vi "MM Sample Test.vi"(8 "error in":errorcluster, 11 "objects IN":T2) -> (0 "error out":errorcluster, 3 "objects OUT":T2)   [LabVIEW 2011]
uses:
  Controls/Class Objects.ctl
  Modules/File/Configuration/Configuration.lvclass
  Modules/Hardware/PID/PID.lvclass
  Modules/Hardware/Power Supply/Power Supply.lvclass
  Modules/Hardware/Mass Flow Controller/Mass Flow Controller.lvclass
  Modules/Hardware/Valve Controller/Valve Controller.lvclass
  Modules/Hardware/Multimeter/Multimeter.lvclass
  Modules/Hardware/Vapour Generator/Vapour Generator.lvclass
  Modules/File/TDMS/TDMS.lvclass
  Modules/Hardware/Aalborg GFC17/Flow Rate.ctl
  Controls/User Interface Action.ctl
  Functional Global Data/Device Params Global.ctl
  Modules/File/TDMS/Data Type.ctl
  Controls/TDMS File Handling.ctl
  Modules/Hardware/Aalborg GFC17/Aalborg GFC17.lvclass
panel:
  in  "MFC Flow Rate":T1 caption="Flow Rate" min=0.0 max=200.0 scale=0.0..200.0
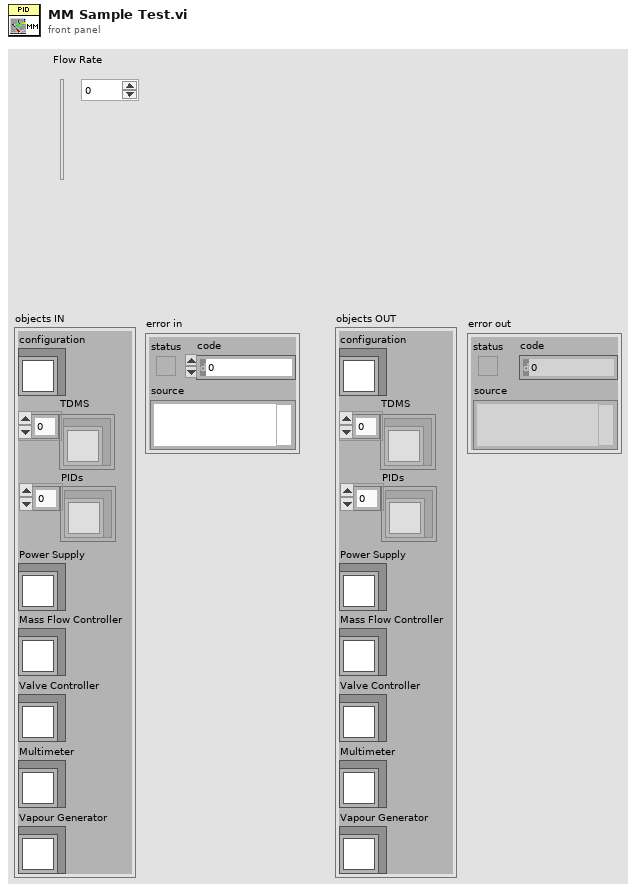
[diagram p1: front panel]
types:
  T1 = typedef "Aalborg GFC17.lvclass/Flow Rate.ctl" = dbl
  T2 = typedef "Class Objects.ctl" = cluster{"configuration":refnum<class "Configuration.lvclass">, "TDMS":refnum<class "TDMS.lvclass">[], "Power Supply":refnum<class "Power Supply.lvclass">, "Mass Flow Controller":refnum<class "Mass Flow Controller.lvclass">, "Valve Controller":refnum<class "Valve Controller.lvclass">, "Multimeter":refnum<class "Multimeter.lvclass">, "Vapour Generator":refnum<class "Vapour Generator.lvclass">, "PIDs":refnum<class "PID.lvclass">[]}
  T3 = typedef "User Interface Action.ctl" = enum16{"Initialize", "Data Acquisition Disable", "Data View Disable", "Sample Set", "Sample Set 2D Data", "Sample Set x0 & dx", "Sample Add", "Sample Set Cursor", "Sample Set Offset & Multiplier", "Sample Set Axis Labels", "Sample Parameters Disabled", "Sample Parameters Update", "Run Update", "Run Set Offset & Multiplier", "Run Set Axis Labels", "Run Set Cursor", "Run Set Disabled", "Run Parameters Update", "Run Parameters Disabled", "Run Number Set", "Run Number Set Range", "Run Number Set Disabled", "Sample Number Set", "Sample Number Set Range", "Notes Set Value", "Update Plot", "Set Plot Parameters", "Update Concentration Plot", "Time Set", "Clear DAQ Display", "Clear Analysis Display", "Status Bar Set", "Progress Bar Set", "Display Mode Set", "Experiment Type Set", "Analysis Plot Average Set", "Stop"}
  T4 = typedef "Device Params Global.ctl" = enum16{"Initialize", "Get Device Settings", "Get Device Connections", "Set Device Settings", "Set Device Connections", "Get All Device Properties"}
  T5 = typedef "TDMS.lvclass/Data Type.ctl" = enum16{"I16", "Double", "Waveform"}
  T6 = typedef "TDMS File Handling.ctl" = enum16{"Add TDMS File", "Get Active TDMS File", "Set Active TDMS File", "Set Active TDMS File Index"}
  T7 = typedef "Device Settings.ctl" = cluster{"PID":cluster{"B-M PID":T8, "INL PID":T9}, "Power Supply":cluster{"Source Value":dbl, "Source Value Units":T10, "Source Mode":T11, "Limits":T12, "Output":bool}, "Mass Flow Controller":cluster{"MFC Flow Rate":dbl, "MFC Valve Status":T15}, "Valve Controller":cluster{"Valve Assembly":T16}, "Multimeter":cluster{"Agilent 3458A":cluster{"Measurement Configuration":T18, "Measurement Integration":T19}}, "Vapour Generator":cluster{"Owlstone Permeation Tube":T20, "Owlstone GEN-SYS Setpoints":T22}}
  T8 = typedef "Baseline Mocon piD-Tech plus.lvclass/Settings.ctl" = cluster{"Detector Sampling Frequency":dbl}
  T9 = typedef "INL PID.lvclass/Settings.ctl" = cluster{"Sampling Frequency":dbl, "Integration Time":dbl, "Integration Periods":u8, "Grid Voltage":dbl}
  T10 = typedef "Power Supply.lvclass/Source Units.ctl" = enum16{"volts", "millivolts", "microvolts", "amps", "milliamps", "microamps", "nanoamps"}
  T11 = typedef "Power Supply.lvclass/Source Mode.ctl" = enum16{"Volts", "Current"}
  T12 = typedef "Power Supply.lvclass/Protection Limits.ctl" = cluster{"Voltage Limit":dbl, "Voltage Limit Units":T13, "Current Limit":dbl, "Current Limit Units":T14, "Voltage Trip/Cmpl":dbl, "Voltage Trip/Cmpl Units":T13, "Current Trip/Cmpl":dbl, "Current Trip/Cmpl Units":T14}
  T13 = typedef "Power Supply.lvclass/Voltage Units.ctl" = enum16{"volts", "millivolts", "microvolts"}
  T14 = typedef "Power Supply.lvclass/Current Units.ctl" = enum16{"amps", "milliamps", "microamps", "nanoamps"}
  T15 = typedef "Mass Flow Controller.lvclass/Valve Status.ctl" = enum16{"Open", "Closed"}
  T16 = typedef "Valve Controller.lvclass/Valve Assembly.ctl" = cluster{"Valve 1":T17, "Valve 2":T17, "Valve 3":T17, "Valve 4":T17, "Valve 5":T17}
  T17 = typedef "Valve Controller.lvclass/Status.ctl" = u16
  T18 = typedef "Agilent 3458A.lvclass/Measurement Configuration.ctl" = cluster{"Function":enum16{"DC Voltage", "AC Voltage", "AC + DC Voltage", "DC Current", "AC Current", "AC + DC Current", "2-Wire Resistance", "4-Wire Resistance", "Frequency", "Period", "Direct Sampling DC", "Direct Sampling AC", "Sub-Sampling DC", "Sub-Sampling AC"}, " Manual Resolution":enum16{"4.5", "5.5", "6.5", "7.5", "8.5"}, "Frequency Source":enum16{"AC + DC Current", "AC + DC Voltage", "AC Current", "AC Voltage"}, "Auto Range":enum16{"OFF", "ON", "ONCE"}}
  T19 = typedef "Agilent 3458A.lvclass/Measurement Integration.ctl" = cluster{"Power Line Cycles":dbl}
  T20 = typedef "Owlstone GEN-SYS.lvclass/Permeation Tube.ctl" = cluster{"Tube":T21, "Molecular Weight":dbl, "Calibration Temperature\n(Celcius)":i32, "Permeation Rate \n(ng/min)":i32}
  T21 = typedef "Owlstone GEN-SYS.lvclass/Permeation Tube Gas.ctl" = enum16{"Isobutylene 27 Nov 2012", "Ammonia 29 Sep 2012", "DMMP Tube A 3 July 2014", "DMMP Tube B 3 July 2014"}
  T22 = typedef "Owlstone GEN-SYS.lvclass/Gen-Sys Setpoints.ctl" = cluster{"OVG-4":cluster{"Oven Temperature":i32, "Sample Flow Rate":i32, "Split Flow Status":u16, "Split Flow Rate":i32}, "OHG-4":cluster{"Wet Air Flow":i32}}
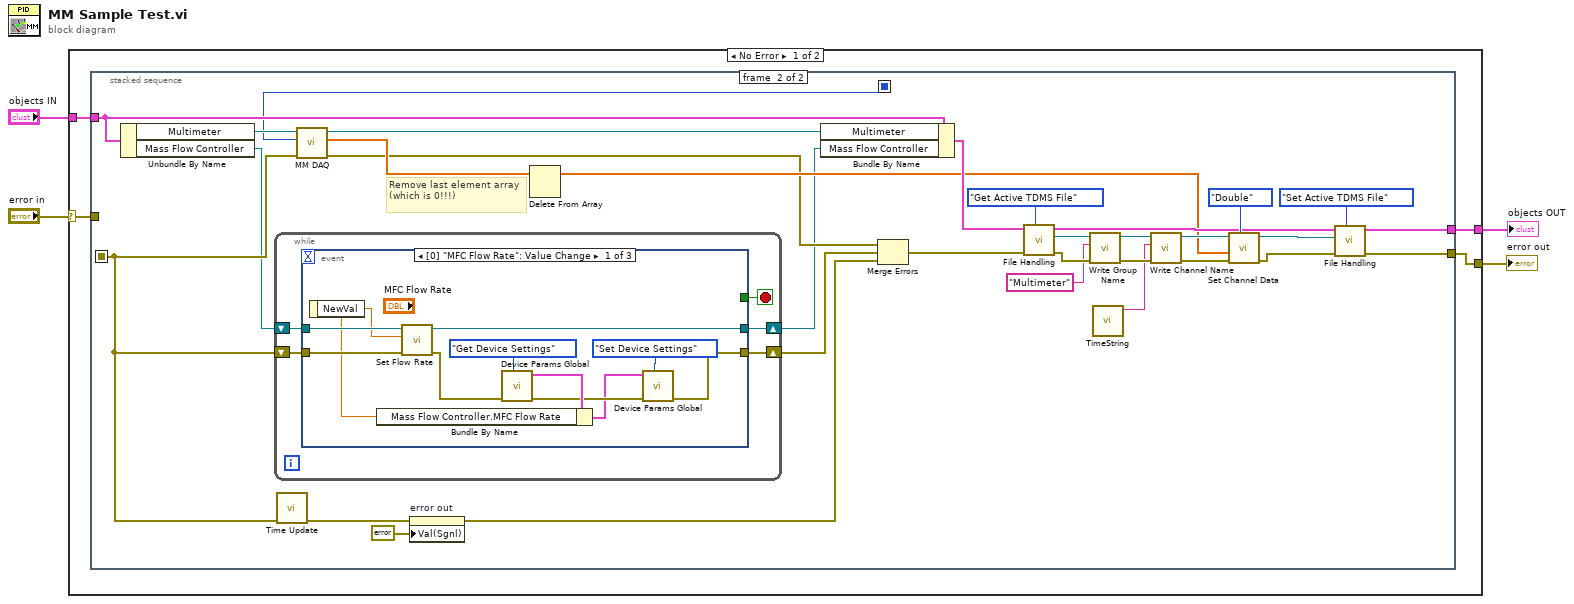
[diagram p0: block diagram]
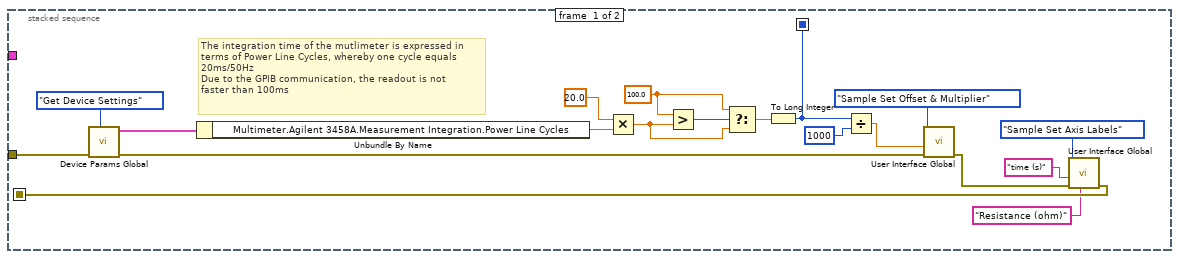
[diagram p2: hidden frame]
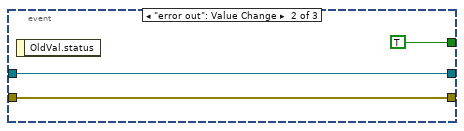
[diagram p3: hidden frame]
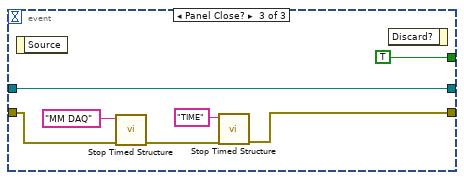
[diagram p4: hidden frame]
diagram:
  n1 = case shown="No Error" "error in" {
    selector: "error in" -> [w5 w86]
    tunnel: "objects IN" -> [w8 w87]
    tunnel: [w6 w87] -> w3
    tunnel: [w7 w86] -> w1
    frame No Error {
      n2 = stacked-sequence {
        seq-local: [w16 _] -> [_ w39]
        seq-local: [w10 _] -> [_ w36]
        tunnel: w8 -> [_ w59]
        tunnel: [_ w52] -> w7
        tunnel: [_ w50] -> w6
        tunnel: w5 -> [w25 _]
        frame #0 {
          w21 = 100.0 ("x")
          # "The integration time of the mutlimeter is expressed in\nterms of Power Line Cycles, whereby one cycle equals\n20ms/50Hz\nDue to the GPIB communication, the readout is not\nfaster than 100ms"
          n3 = call "Device Params Global.vi"("action"=Device_Params_Global."Get Device Settings", "error in"=w25) -> ("error out"=w17:errorcluster, "Device Settings OUT"=w26:T7)  [unwired: 7 in, 1 out]
          n4 = Unbundle By Name(w26) -> ("Multimeter.Agilent 3458A.Measurement Integration.Power Line Cycles"=w24:dbl)
          n5 = Multiply(x=20.0, y=w24) -> (x*y=w20:dbl)
          n6 = Greater?(x=w21, y=w20) -> (0:w22:bool)
          n7 = Select(t=w21, s=w22, f=w20) -> (s? t:f=w19:dbl)
          n8 = To Long Integer(number=w19) -> (32bit integer=w16:i32)
          n9 = Divide(x=w16, y=1000) -> (x/y=w14:dbl)
          n10 = call "User Interface Global.vi"("error in"=w17, "data1"=w14, "action"=User_Interface_Action."Sample Set Offset & Multiplier") -> ("error out"=w12:errorcluster)  [unwired: 8 in]
          n11 = call "User Interface Global.vi"("data2"="Resistance (ohm)", "error in"=w12, "data1"="time (s)", "action"=User_Interface_Action."Sample Set Axis Labels") -> ("error out"=w10:errorcluster)  [unwired: 7 in]
        }
        frame #1 {
          # "Remove last element array (which is 0!!!)"
          n12 = Unbundle By Name(w59) -> ("Multimeter"=w41:refnum<class "Multimeter.lvclass">, "Mass Flow Controller"=w35:refnum<class "Mass Flow Controller.lvclass">)
          n13 = while {
            shift-right: [w60] -> w32
            shift-left: w35 -> [w64]
            shift-right: [w62] -> w31
            shift-left: w36 -> [w63]
            stop <- w61 stop-if-true
            n14 = event shown="[0] \"MFC Flow Rate\": Value Change" {
              selector: _ -> [_ _ _]
              dyn-events: _ -> [_ _ _]
              timeout: _ -> [_ _ _]
              tunnel: w64 -> [w75 w76 w84]
              tunnel: w63 -> [w74 w77 w85]
              tunnel: [w73 w76 w84] -> w60
              tunnel: [w65 w77 w80] -> w62
              tunnel: [_ TRUE TRUE] -> w61
              event Value Change {
                n15 = event-data() -> ("NewVal"=w70:T1)  [unwired: 1 in]
                n16 = call-dynamic "Set Flow Rate.vi"("error in (no error)"=w74, "Flow Rate"=w70, "Mass Flow Controller in"=w75) -> ("error out"=w69:errorcluster, "Mass Flow Controller out"=w73:refnum<class "Mass Flow Controller.lvclass">)  [unwired: 7 in]
                n17 = call "Device Params Global.vi"("action"=Device_Params_Global."Get Device Settings", "error in"=w69) -> ("error out"=w67:errorcluster, "Device Settings OUT"=w71:T7)  [unwired: 7 in, 1 out]
                n18 = Bundle By Name(cluster=w71, "Mass Flow Controller.MFC Flow Rate"=w70) -> (w66:T7)
                n19 = call "Device Params Global.vi"("action"=Device_Params_Global."Set Device Settings", "error in"=w67, "Device Settings IN"=w66) -> ("error out"=w65:errorcluster)  [unwired: 6 in, 2 out]
              }
              event "error out": Value Change {
                n20 = event-data() -> ()  [unwired: 1 in, 1 out]
              }
              event Panel Close? {
                n21 = event-data() -> ()  [unwired: 1 in, 1 out]
                n22 = call <vilib>:"Stop Timed Structure.vi"("error in (no error)"=w85, "name"="MM DAQ") -> ("error out"=w81:errorcluster)  [unwired: 9 in]
                n23 = call <vilib>:"Stop Timed Structure.vi"("error in (no error)"=w81, "name"="TIME") -> ("error out"=w80:errorcluster)  [unwired: 9 in]
                n24 = event-data() -> ()  [unwired: 2 in, 1 out]
              }
            }
          }
          n25 = call "Time Update.vi"("error in"=w36) -> ("error out"=w30:errorcluster)  [unwired: 10 in]
          n26 = call "MM DAQ.vi"("error in"=w36, "DAQ dt"=w39, "Multimeter in"=w41) -> ("error out"=w33:errorcluster, "Data"=w38:dbl[], "Multimeter out"=w40:refnum<class "Multimeter.lvclass">)  [unwired: 6 in]
          n27 = property on="error out" class="Clust (strict)"(error in=w30, "Val(Sgnl)"=errorcluster {"status"=FALSE, "code"=0, "source"=""} ("Value (Signaling)")) -> (error out=w28:errorcluster)  [unwired: 1 in, 1 out]
          n28 = Delete From Array(array=w38) -> (array with subset deleted=w37:dbl[])  [unwired: 2 in, 1 out]
          n29 = Bundle By Name(cluster=w59, "Multimeter"=w40, "Mass Flow Controller"=w32) -> (w57:T2)
          n30 = Merge Errors(w33, w31, w28) -> (w34:errorcluster)
          n31 = call "File Handling.vi"("TDMS File Handling"=TDMS_File_Handling."Get Active TDMS File", "error in"=w34, "Class objects"=w57) -> ("error out"=w48:errorcluster, "TDMS File"=w49:refnum<class "TDMS.lvclass">, "Class objects"=w51:T2)  [unwired: 6 in]
          n32 = call-dynamic "Write Group Name.vi"("error in (no error)"=w48, "Group Name"="Multimeter", "TDMS in"=w49) -> ("error out"=w45:errorcluster, "TDMS out"=w46:refnum<class "TDMS.lvclass">)  [unwired: 7 in]
          n33 = call "TimeString.vi"() -> ("String"=w42:string)  [unwired: 11 in]
          n34 = call-dynamic "Write Channel Name.vi"("error in (no error)"=w45, "Channel Name"=w42, "TDMS in"=w46) -> ("error out"=w44:errorcluster, "TDMS out"=w43:refnum<class "TDMS.lvclass">)  [unwired: 7 in]
          n35 = call-dynamic "Set Channel Data.vi"("data type"=Data_Type."Double", "error in"=w44, "double channel data"=w37, "TDMS in"=w43) -> ("error out"=w53:errorcluster, "TDMS out"=w55:refnum<class "TDMS.lvclass">)  [unwired: 6 in]
          n36 = call "File Handling.vi"("TDMS File Handling"=TDMS_File_Handling."Set Active TDMS File", "error in"=w53, "TDMS File"=w55, "Class objects"=w51) -> ("error out"=w52:errorcluster, "Class objects"=w50:T2)  [unwired: 5 in, 1 out]
        }
      }
    }
    frame Error {
    }
  }
  "objects OUT" <- w3
  "error out" <- w1
